vi "ControlDriveMotors.vi"(1 "Braking":bool, 2 "Robot Motion Commands":T1) -> ()   [LabVIEW 2019]
uses:
  Controls/Robot Pivot Motion Commands.ctl
  Controls/Pivot Motor Commands.ctl
  Controls/Robot Drive Mode.ctl
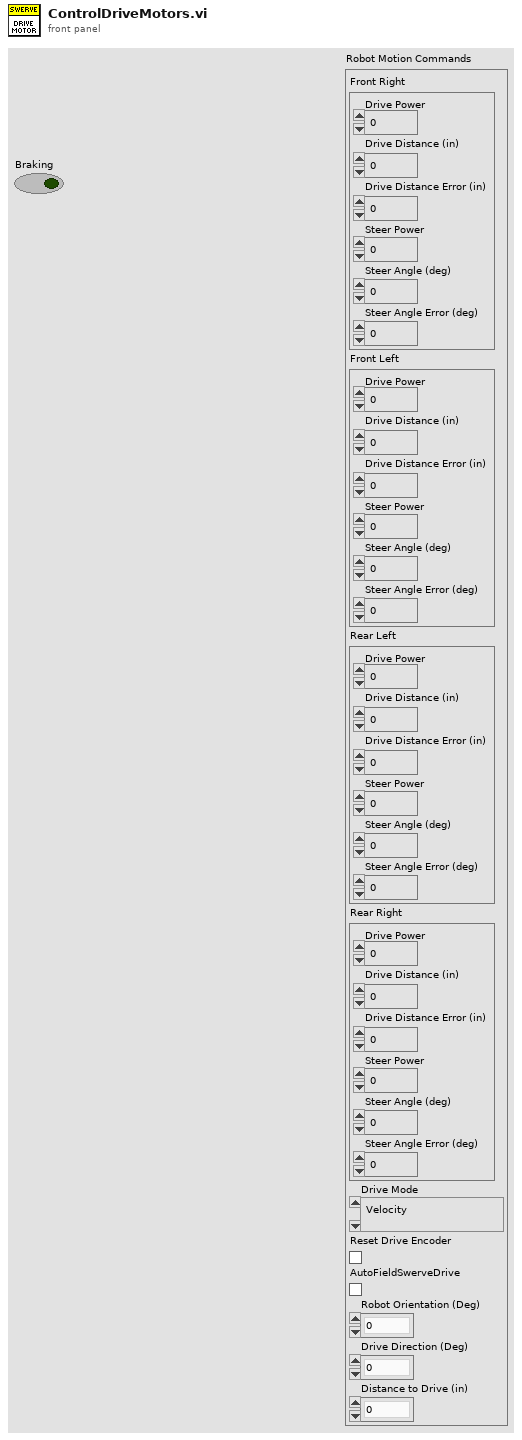
[diagram p1: front panel]
types:
  T1 = typedef "Robot Pivot Motion Commands.ctl" = cluster{"Front Right":T2, "Front Left":T2, "Rear Left":T2, "Rear Right":T2, "Drive Mode":T3, "Reset Drive Encoder":bool, "AutoFieldSwerveDrive":bool, "Robot Orientation (Deg)":dbl, "Drive Direction (Deg)":dbl, "Distance to Drive (in)":dbl}
  T2 = typedef "Pivot Motor Commands.ctl" = cluster{"Drive Power":dbl, "Drive Distance (in)":dbl, "Drive Distance Error (in)":dbl, "Steer Power":dbl, "Steer Angle (deg)":dbl, "Steer Angle Error (deg)":dbl}
  T3 = typedef "Robot Drive Mode.ctl" = enum16{"Velocity", "Distance"}
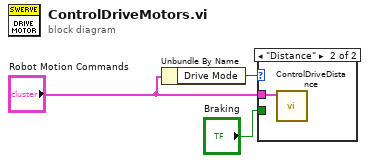
[diagram p0: block diagram]
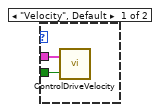
[diagram p2: hidden frame]
diagram:
  n1 = Unbundle By Name("Robot Motion Commands") -> ("Drive Mode"=w3:T3)
  n2 = case shown="\"Distance\"" w3 {
    tunnel: "Robot Motion Commands" -> [w5 w6]
    tunnel: "Braking" -> [w4 _]
    frame "Velocity", Default {
      n3 = call "ControlDriveVelocity.vi"("Braking"=w4, "Robot Motion Commands"=w5) -> ()  [unwired: 1 in]
    }
    frame "Distance" {
      n4 = call "ControlDriveDistance.vi"("Robot Motion Commands"=w6) -> ()  [unwired: 11 in]
    }
  }
